vi "oldArduinoMicro Module.vi"(5 "Enable":bool=TRUE, 6 "Timeout(s)":dbl=2.0, 7 "Command":T3, 8 "error in (no error)":errorcluster, 10 "VALVES":T1, 11 "VISA resource name":refnum<visa-resource-name>="COM39") -> (0 "error out":errorcluster, 1 "Output":T2, 2 "read string":string, 3 "TimeOut":bool, 4 "write string":string)   [LabVIEW 2013]
uses:
  ArduinoMicro Module Control.ctl
  <vilib>/Instr/_visa.llb/VISA Configure Serial Port (Instr).vi
panel:
  out "Bytes at Serial Port 2":u32
  out "Bytes at Serial Port":u32
  out "read string 2":string
  # "Output Data"
  # "Input Data"
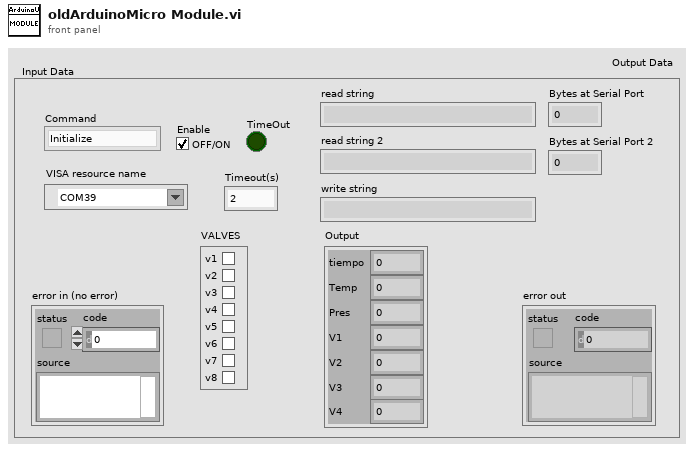
[diagram p1: front panel]
types:
  T1 = cluster{"v1":bool, "v2":bool, "v3":bool, "v4":bool, "v5":bool, "v6":bool, "v7":bool, "v8":bool}
  T2 = cluster{"tiempo":dbl, "Temp":dbl, "Pres":dbl, "V1":dbl, "V2":dbl, "V3":dbl, "V4":dbl}
  T3 = typedef "ArduinoMicro Module Control.ctl" = enum16{"Initialize", "Read Data", "Write Data", "Enable", "Disable", "Shutdown"}
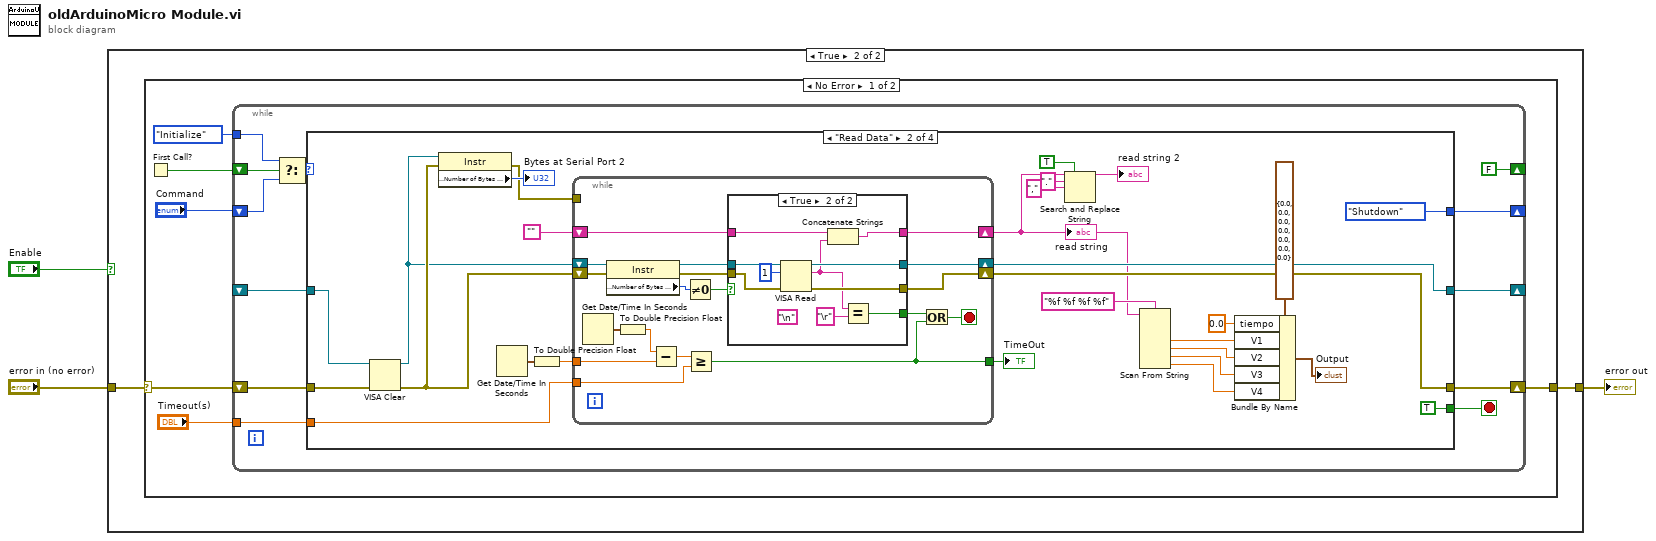
[diagram p0: block diagram]
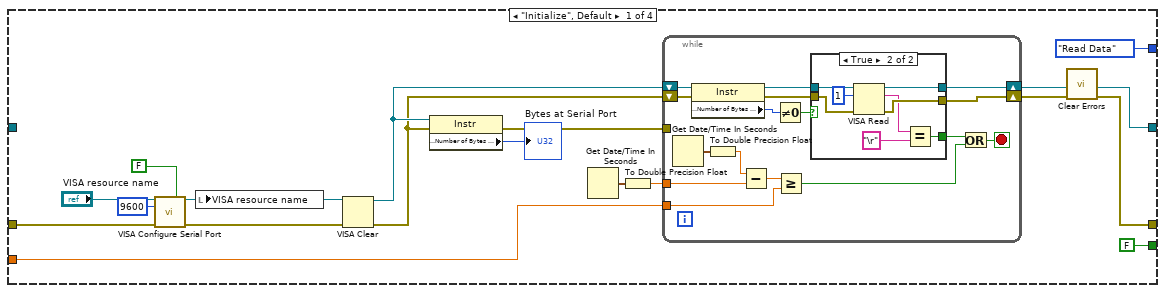
[diagram p3: hidden frame]
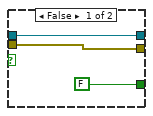
[diagram p4: hidden frame]
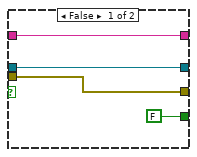
[diagram p5: hidden frame]
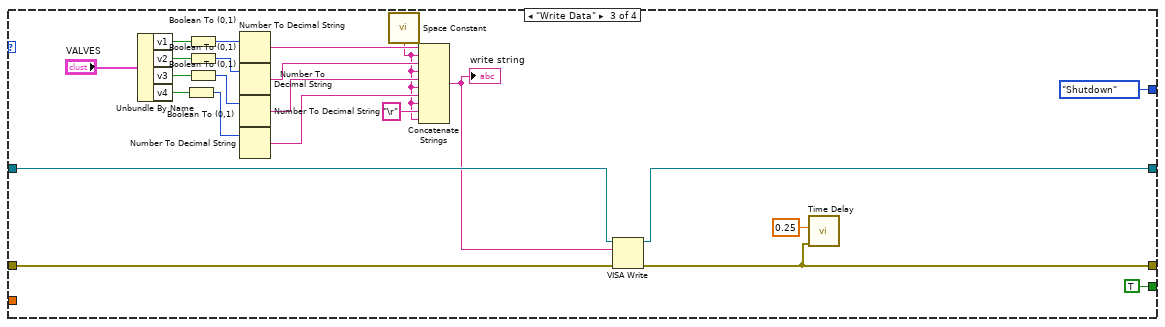
[diagram p6: hidden frame]
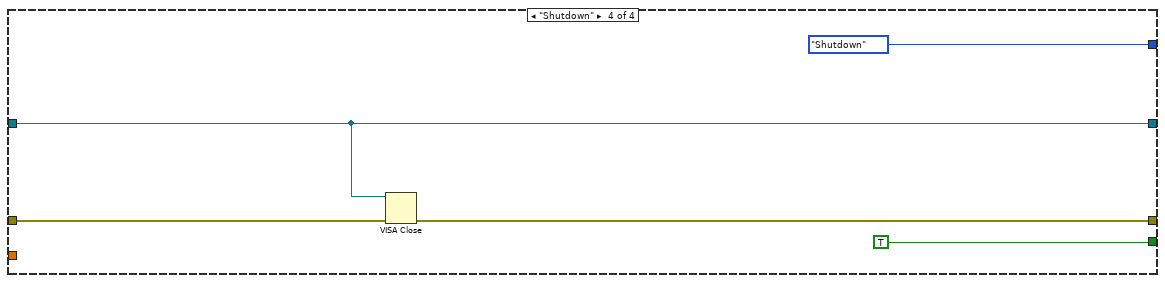
[diagram p7: hidden frame]
diagram:
  n1 = case shown="True" "Enable" {
    tunnel: "error in (no error)" -> [w4 w6]
    tunnel: [w4 w5] -> w2
    frame False {
    }
    frame True {
      n2 = case shown="No Error" w6 {
        selector: w6 -> [w10 w158]
        tunnel: [w9 w158] -> w5
        frame No Error {
          n3 = First Call?() -> (First Call?: T/F=w12:bool)
          n4 = while {
            shift-right: [w15] -> _
            shift-left: "Command" -> [w21]
            shift-right: [w18] -> w9
            shift-left: w10 -> [w19]
            shift-right: [FALSE ("First Call?: T/F")] -> _
            shift-left: w12 -> [w24]
            tunnel: ArduinoMicro_Module_Control."Initialize" ("t") -> [w23]
            shift-right: [w17] -> _
            shift-left: _ -> [w16]
            tunnel: "Timeout(s)" -> [w13]
            stop <- w14 stop-if-true
            n5 = Select(t=w23, s=w24, f=w21) -> (s? t:f=w20:T3)
            n6 = case shown="\"Read Data\"" w20 {
              tunnel: w19 -> [w37 w78 w152 w154]
              tunnel: [w26 w89 w130 w153] -> w18
              tunnel: [w33 w90 w149 w155] -> w17
              tunnel: w16 -> [_ w76 w148 w155]
              tunnel: [ArduinoMicro_Module_Control."Read Data" ("t") ArduinoMicro_Module_Control."Shutdown" ("t") ArduinoMicro_Module_Control."Shutdown" ("t") ArduinoMicro_Module_Control."Shutdown" ("t")] -> w15
              tunnel: [FALSE ("Enable Termination\nChar (T)") TRUE ("Enable Termination\nChar (T)") TRUE ("Enable Termination\nChar (T)") TRUE ("Enable Termination\nChar (T)")] -> w14
              tunnel: w13 -> [w32 w93 _ _]
              frame "Initialize", Default {
                n7 = call-poly "VISA Configure Serial Port"("VISA resource name"="VISA resource name", "Enable Termination\nChar (T)"=FALSE ("Enable Termination\nChar (T)"), "baud rate (9600)"=u32 9600, "error in (no error)"=w37) -> ("VISA resource name out"=w31:refnum<visa-resource-name>, "error out"=w30:errorcluster)  [unwired: 10 in]
                n8 = local write "VISA resource name"(w31) -> ()
                n9 = VISA Clear(VISA resource name=w31, error in (no error)=w30) -> (VISA resource name out=w29:refnum<visa-resource-name>, error out=w28:errorcluster)
                n10 = property class="Instr"(reference=w29, error in=w28) -> (error out=w25:errorcluster, "Serial Settings:Number of Bytes at Serial Port"=→"Bytes at Serial Port":u32)  [unwired: 1 out]
                n11 = Get Date/Time In Seconds() -> (seconds since 1Jan1904=w36:timestamp)
                n12 = To Double Precision Float(number=w36) -> (double precision float=w35:dbl)
                n13 = while {
                  tunnel: w35 -> [w43]
                  shift-right: [w53] -> w33
                  shift-left: w29 -> [w51]
                  shift-right: [w52] -> w34
                  shift-left: w28 -> [w50]
                  tunnel: w32 -> [w44]
                  tunnel: w25 -> [_]
                  stop <- w58 stop-if-true
                  n14 = Get Date/Time In Seconds() -> (seconds since 1Jan1904=w57:timestamp)
                  n15 = property class="Instr"(reference=w51, error in=w50) -> (reference out=w48:refnum<visa-resource-name>, error out=w49:errorcluster, "Serial Settings:Number of Bytes at Serial Port"=w47:u32)
                  n16 = To Double Precision Float(number=w57) -> (double precision float=w56:dbl)
                  n17 = Subtract(x=w56, y=w43) -> (x-y=w55:dbl)
                  n18 = Not Equal To 0?(x=w47) -> (x != 0?=w46:bool)
                  n19 = Greater Or Equal?(x=w55, y=w44) -> (x >= y?=w54:bool)
                  n20 = case shown="True" w46 {
                    tunnel: [w61 w69] -> w53
                    tunnel: [w60 w68] -> w52
                    tunnel: w49 -> [w60 w67]
                    tunnel: w48 -> [w61 w66]
                    tunnel: [FALSE w63] -> w45
                    frame False {
                    }
                    frame True {
                      n21 = VISA Read(VISA resource name=w66, byte count=u32 1, error in (no error)=w67) -> (VISA resource name out=w69:refnum<visa-resource-name>, read buffer=w64:string, error out=w68:errorcluster)  [unwired: 1 out]
                      n22 = Equal?(x=w64, y="\r" ("Mide")) -> (x = y?=w63:bool)
                    }
                  }
                  n23 = Or(x=w45, y=w54) -> (x .or. y?=w58:bool)
                }
                n24 = call <vilib>:"Clear Errors.vi"("error in (no error)"=w34) -> ("error out"=w26:errorcluster)  [unwired: 6 in]
              }
              frame "Read Data" {
                n25 = VISA Clear(VISA resource name=w76, error in (no error)=w78) -> (VISA resource name out=w75:refnum<visa-resource-name>, error out=w77:errorcluster)
                n26 = property class="Instr"(reference=w75, error in=w77) -> (error out=w74:errorcluster, "Serial Settings:Number of Bytes at Serial Port"=→"Bytes at Serial Port 2":u32)  [unwired: 1 out]
                n27 = Get Date/Time In Seconds() -> (seconds since 1Jan1904=w92:timestamp)
                n28 = To Double Precision Float(number=w92) -> (double precision float=w91:dbl)
                n29 = while {
                  tunnel: w91 -> [w112]
                  shift-right: [w108] -> w90
                  shift-left: w75 -> [w106]
                  shift-right: [w107] -> w89
                  shift-left: w77 -> [w105]
                  tunnel: w93 -> [w110]
                  tunnel: [w109] -> w94
                  shift-right: [w99] -> w73
                  shift-left: "" -> [w100]
                  tunnel: w74 -> [_]
                  stop <- w115 stop-if-true
                  n30 = Get Date/Time In Seconds() -> (seconds since 1Jan1904=w114:timestamp)
                  n31 = property class="Instr"(reference=w106, error in=w105) -> (reference out=w103:refnum<visa-resource-name>, error out=w104:errorcluster, "Serial Settings:Number of Bytes at Serial Port"=w102:u32)
                  n32 = To Double Precision Float(number=w114) -> (double precision float=w113:dbl)
                  n33 = Subtract(x=w113, y=w112) -> (x-y=w111:dbl)
                  n34 = Not Equal To 0?(x=w102) -> (x != 0?=w101:bool)
                  n35 = Greater Or Equal?(x=w111, y=w110) -> (x >= y?=w109:bool)
                  n36 = case shown="True" w101 {
                    tunnel: [w119 w129] -> w108
                    tunnel: [w118 w128] -> w107
                    tunnel: w104 -> [w118 w127]
                    tunnel: w103 -> [w119 w126]
                    tunnel: w100 -> [w117 w125]
                    tunnel: [w117 w124] -> w99
                    tunnel: [FALSE w121] -> w98
                    frame False {
                    }
                    frame True {
                      (unwired) "\n"
                      n37 = VISA Read(VISA resource name=w126, byte count=u32 1, error in (no error)=w127) -> (VISA resource name out=w129:refnum<visa-resource-name>, read buffer=w122:string, error out=w128:errorcluster)  [unwired: 1 out]
                      n38 = Concatenate Strings(w125, w122) -> (w124:string)
                      n39 = Equal?(x=w122, y="\r" ("Mide")) -> (x = y?=w121:bool)
                    }
                  }
                  n40 = Or(x=w98, y=w109) -> (x .or. y?=w115:bool)
                }
                "read string" <- w73
                "TimeOut" <- w94
                n41 = Search and Replace String(replace all?=TRUE ("replace all? (F)"), input string=w73, search string=".", replace string="," ("replace string (\"\")")) -> (result string=→"read string 2":string)  [unwired: 4 in, 3 out]
                n42 = Scan From String(format string="%f %f %f %f", input string=w73) -> (output 1=w71:dbl, output 2=w70:dbl, output 3=w87:dbl, output 4=w86:dbl)  [unwired: 6 in, 3 out]
                n43 = Bundle By Name(cluster=T2 {"tiempo"=0.0, "Temp"=0.0, "Pres"=0.0, "V1"=0.0, "V2"=0.0, "V3"=0.0, "V4"=0.0} ("Output"), "tiempo"=0.0, "V1"=w71, "V2"=w70, "V3"=w87, "V4"=w86) -> (→"Output":T2)
              }
              frame "Write Data" {
                n44 = Unbundle By Name("VALVES") -> ("v1"=w146:bool, "v2"=w145:bool, "v3"=w144:bool, "v4"=w143:bool)
                n45 = Boolean To (0,1)(Boolean=w143) -> (0, 1=w138:i16)
                n46 = Boolean To (0,1)(Boolean=w146) -> (0, 1=w142:i16)
                n47 = Boolean To (0,1)(Boolean=w145) -> (0, 1=w140:i16)
                n48 = Boolean To (0,1)(Boolean=w144) -> (0, 1=w139:i16)
                n49 = Number To Decimal String(number=w142) -> (decimal integer string=w141:string)  [unwired: 1 in]
                n50 = Number To Decimal String(number=w140) -> (decimal integer string=w137:string)  [unwired: 1 in]
                n51 = Number To Decimal String(number=w139) -> (decimal integer string=w136:string)  [unwired: 1 in]
                n52 = Number To Decimal String(number=w138) -> (decimal integer string=w135:string)  [unwired: 1 in]
                n53 = call <vilib>:"Space Constant.vi"() -> ("String"=w132:string)
                n54 = Concatenate Strings(w141, w132, w137, w132, w136, w132, w135, w132, "\r" ("string"), w132) -> (w133:string)
                "write string" <- w133
                n55 = VISA Write(VISA resource name=w148, write buffer=w133, error in (no error)=w152) -> (VISA resource name out=w149:refnum<visa-resource-name>, error out=w130:errorcluster)  [unwired: 1 out]
                n56 = call "Time Delay"("error in (no error)"=w130, "Delay Time (s)"=0.25) -> ()  [unwired: 9 in, 1 out]
              }
              frame "Shutdown" {
                n57 = VISA Close(VISA resource name=w155, error in (no error)=w154) -> (error out=w153:errorcluster)
              }
            }
          }
        }
        frame Error {
        }
      }
    }
  }
  "error out" <- w2
